vi "Edit Build CHM CFG File Title Key.vi"(8 "error in":errorcluster, 9 "CD name":string, 10 "relative path of CFG file to edit":path, 11 "custom device path":path) -> (0 "error out":errorcluster, 3 "custom device path out":path)   [LabVIEW 2020, in "Template Tool.lvlib"]
uses:
  Template Tool.lvlib
  <vilib>/Utility/config.llb/Write Key (String).vi
  <vilib>/Utility/config.llb/NI_LVConfig.lvlib
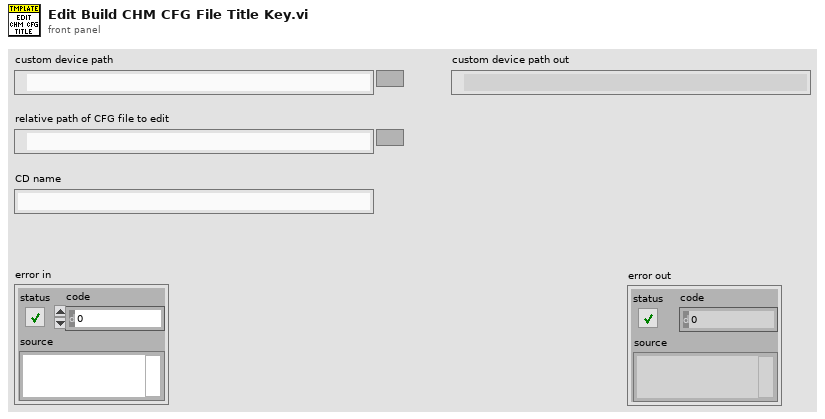
[diagram p1: front panel]
types:
  T1 = typedef "NI_LVConfig.lvlib/Config Data RefNum.ctl" = refnum<k1>
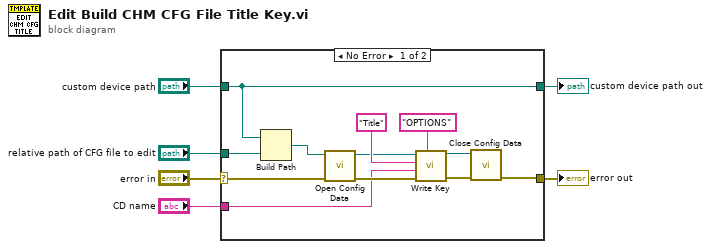
[diagram p0: block diagram]
diagram:
  n1 = case shown="No Error" "error in" {
    selector: "error in" -> [w13 w19]
    tunnel: [w8 w19] -> w6
    tunnel: "custom device path" -> [w17 w20]
    tunnel: "relative path of CFG file to edit" -> [w18 _]
    tunnel: [w17 w20] -> w3
    tunnel: "CD name" -> [w7 _]
    frame No Error {
      n2 = Build Path(base path=w17, name or relative path=w18) -> (appended path=w12:path)
      n3 = call <vilib>:"Open Config Data.vi"("error in (no error)"=w13, "configuration file path"=w12) -> ("error out"=w15:errorcluster, "refnum"=w14:T1)  [unwired: 7 in, 1 out]
      n4 = call-poly <vilib>:"Write Key.vi"("section"="OPTIONS", "error in (no error)"=w15, "value"=w7, "key"="Title", "refnum"=w14) -> ("error out"=w10:errorcluster, "refnum out"=w9:T1)  [unwired: 4 in, 1 out]
      n5 = call <vilib>:"Close Config Data.vi"("error in (no error)"=w10, "refnum"=w9) -> ("error out"=w8:errorcluster)  [unwired: 8 in, 1 out]
    }
    frame Error {
    }
  }
  "error out" <- w6
  "custom device path out" <- w3
